vi "Update_Mapping_GBL.vi"(9 "angles[]":dbl[](array[numeric]), 10 "distance[]":dbl[](array[numeric]), 11 "Current_Position_out":T1) -> ()   [LabVIEW 2017]
uses:
  Ctl/Current_Position.ctl
  Mapping_GBL.vi
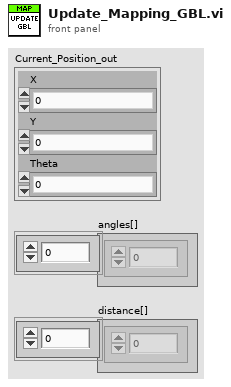
[diagram p1: front panel]
types:
  T1 = typedef "Current_Position.ctl" = cluster{"X":dbl, "Y":dbl, "Theta":dbl}
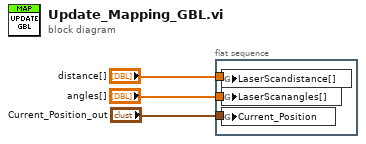
[diagram p0: block diagram]
diagram:
  n1 = flat-sequence {
    tunnel: "Current_Position_out" -> [w6]
    tunnel: "distance[]" -> [w4]
    tunnel: "angles[]" -> [w5]
    frame #0 {
      n2 = global write "Mapping_GBL.vi" "LaserScandistance[]"(w4) -> ()
      n3 = global write "Mapping_GBL.vi" "LaserScanangles[]"(w5) -> ()
      n4 = global write "Mapping_GBL.vi" "Current_Position"(w6) -> ()
    }
  }
